vi "Write Input Filter.vi"(8 "error in (no error)":errorcluster, 10 "Input Filter":u32(ring)=128 items=["1 us"=0, "16 us"=1, "256 us"=2, "4096 us"=3, "Disabled"=128], 11 "SD Module in":refnum<class "SD Module.lvclass">) -> (0 "error out":errorcluster, 3 "SD Module out":refnum<class "SD Module.lvclass">)   [LabVIEW 2019, in "Modules.lvlib" / "SD Module.lvclass"]
uses:
  SD Module.lvclass
  SD Module.lvclass/SD Module.ctl
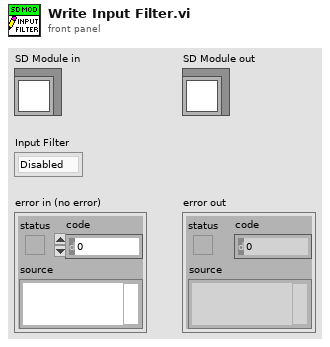
[diagram p1: front panel]
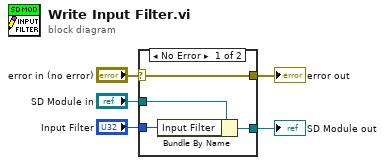
[diagram p0: block diagram]
diagram:
  n1 = case shown="No Error" "error in (no error)" {
    selector: "error in (no error)" -> [w9 w10]
    tunnel: [w9 w10] -> w4
    tunnel: [w7 w11] -> w2
    tunnel: "SD Module in" -> [w8 w11]
    tunnel: "Input Filter" -> [w6 _]
    frame No Error {
      n2 = Bundle By Name(cluster=w8, "Input Filter"=w6) -> (w7:refnum<class "SD Module.lvclass">)
    }
    frame Error {
    }
  }
  "error out" <- w4
  "SD Module out" <- w2
